vi "Loop Counter Timer.vi"(4 "Gate Reset":bool=TRUE, 5 "Trigger Direction":enum8{"either", "false-true", "true-false"}(ring), 6 "Reset":bool, 7 "Waveform":bool) -> (0 "Clock Reset":bool, 1 "Loop Counter":u64, 2 "Ticks Per Loop":u32, 3 "Last Interval between Resets":u64)   [LabVIEW 2009]
doc: "This vi has a multipurpose function. It aacts as a free running timer, which resets to 0 when you send a \"true\" value to the reset input. You can also send a digital signal to the waveform input, and use the \"trigger direction\" input to decide whether to reset the timer on the rising edge, falling edge, or either edge of the waveform input. \n\nThe output terminals show a \"triggered\" boolean, to display if the clock was reset. \"Loop count\" displays the value fo the free-running counter, and increases by 1 with each clock tick. I guess that it resets with size overflows. \"Reset Interval\" measures the time from the last reset to the current one. \"Loop Duration\" tells how many ticks it took to execute the loop. \"Triggered\" outputs true on the tick where the clock was reset"
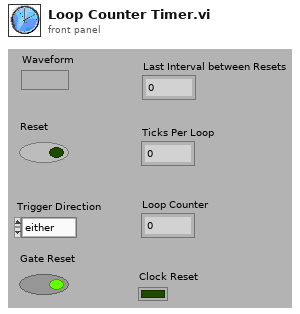
[diagram p1: front panel]
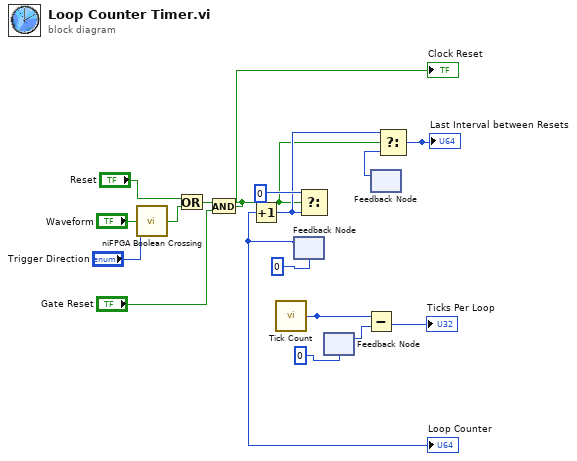
[diagram p0: block diagram]
diagram:
  n1 = call <vilib>:"niFPGA Boolean Crossing.vi"("input"="Waveform", "direction"="Trigger Direction") -> ("crossing"=w7:bool)  [unwired: 1 in, 6 out]
  n2 = Or(x="Reset", y=w7) -> (x .or. y?=w3:bool)
  n3 = And(x=w3, y="Gate Reset") -> (x .and. y?=w2:bool)
  "Clock Reset" <- w2
  n4 = call "Tick Count"() -> ("Tick Count(Ticks)"=w16:u32)
  n5 = feedback #1(u64 0) -> (w8:u64)
  "Loop Counter" <- w8
  n6 = Increment(x=w8) -> (x+1=w9:u64)
  n7 = Select(t=u64 0, s=w2, f=w9) -> (s? t:f=w13:u64)
  n8 = feedback #2(u32 0) -> (w17:u32)
  n9 = Subtract(x=w16, y=w17) -> (x-y=→"Ticks Per Loop":u32)
  n10 = feedback #3() -> (w10:u64)  [unwired: 1 out]
  n11 = Select(t=w9, s=w2, f=w10) -> (s? t:f=w11:u64)
  "Last Interval between Resets" <- w11
